vi "Write File Path.vi"(8 "error in (no error)":errorcluster, 10 "File Path":path, 11 "Log Open Message in":refnum<class "Log Open Message.lvclass">) -> (0 "error out":errorcluster, 3 "Log Open Message out":refnum<class "Log Open Message.lvclass">)   [LabVIEW 2017, in "Messaging.lvlib" / "Log Open Message.lvclass"]
uses:
  Log Open Message.lvclass
  Log Open Message.lvclass/Log Open Message.ctl
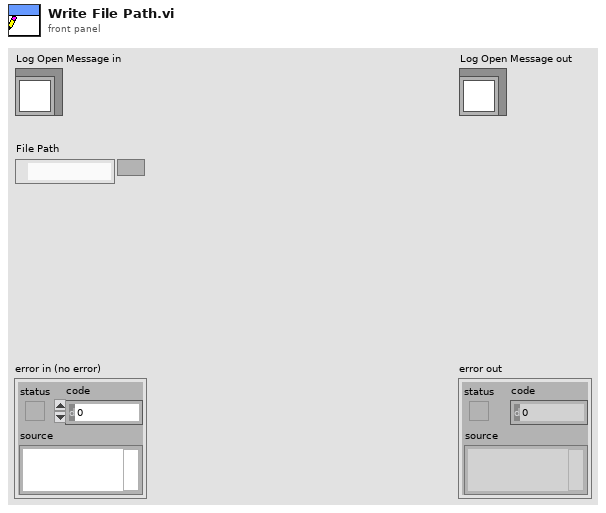
[diagram p1: front panel]
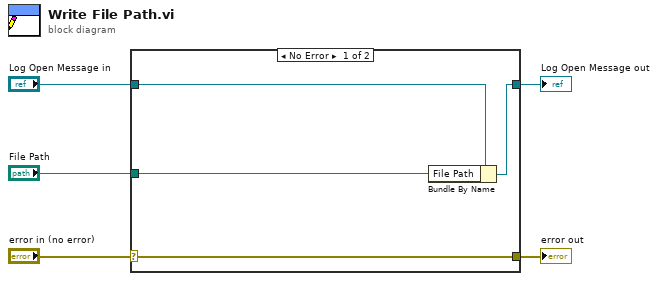
[diagram p0: block diagram]
diagram:
  n1 = case shown="No Error" "error in (no error)" {
    selector: "error in (no error)" -> [w9 w10]
    tunnel: [w9 w10] -> w4
    tunnel: [w7 w11] -> w2
    tunnel: "Log Open Message in" -> [w8 w11]
    tunnel: "File Path" -> [w6 _]
    frame No Error {
      n2 = Bundle By Name(cluster=w8, "File Path"=w6) -> (w7:refnum<class "Log Open Message.lvclass">)
    }
    frame Error {
    }
  }
  "error out" <- w4
  "Log Open Message out" <- w2
